vi "case_simple.vi"() -> ()   [LabVIEW 2021]
panel:
  in  "Enum":enum16{"Plus", "Minus", ""}(ring)
  in  "Numeric 13":dbl
  in  "String":string
  out "Numeric 12":dbl
  in  "Numeric 11":dbl
  in  "Numeric 10":dbl
  out "Numeric 9":dbl
  in  "Numeric 8":dbl
  in  "Numeric 7":dbl
  out "Numeric 6":dbl
  in  "Numeric 5":dbl
  in  "Numeric 4":dbl
  in  "Boolean":bool
  out "Numeric 3":dbl
  in  "Numeric 2":dbl
  in  "Numeric":dbl
  # "Method 1"
  # "Method 2"
  # "Method 3"
  # "Method 4"
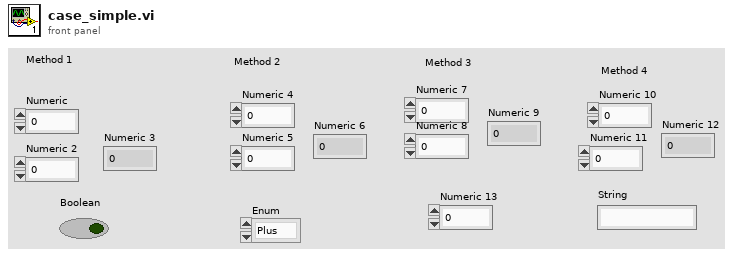
[diagram p1: front panel]
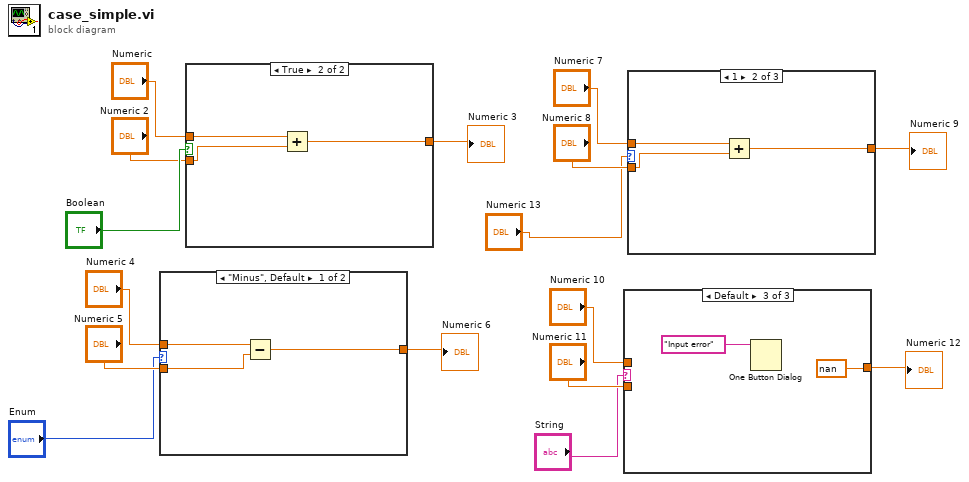
[diagram p0: block diagram]
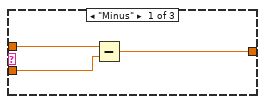
[diagram p2: hidden frame]
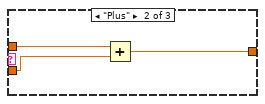
[diagram p3: hidden frame]
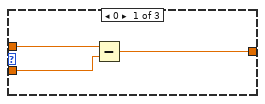
[diagram p4: hidden frame]
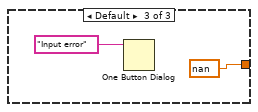
[diagram p5: hidden frame]
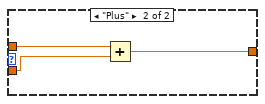
[diagram p6: hidden frame]
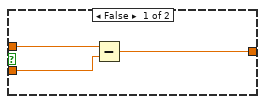
[diagram p7: hidden frame]
diagram:
  n1 = case shown="\"Minus\", Default" "Enum" {
    tunnel: [w19 w22] -> w12
    tunnel: "Numeric 4" -> [w18 w21]
    tunnel: "Numeric 5" -> [w17 w20]
    frame "Minus", Default {
      n2 = Subtract(x=w18, y=w17) -> (x-y=w19:dbl)
    }
    frame "Plus" {
      n3 = Add(x=w21, y=w20) -> (x+y=w22:dbl)
    }
  }
  "Numeric 6" <- w12
  n4 = case shown="True" "Boolean" {
    tunnel: [w25 w28] -> w15
    tunnel: "Numeric" -> [w24 w27]
    tunnel: "Numeric 2" -> [w23 w26]
    frame False {
      n5 = Subtract(x=w24, y=w23) -> (x-y=w25:dbl)
    }
    frame True {
      n6 = Add(x=w27, y=w26) -> (x+y=w28:dbl)
    }
  }
  "Numeric 3" <- w15
  n7 = case shown="Default" "String" {
    tunnel: [w31 w34 nan] -> w6
    tunnel: "Numeric 10" -> [w30 w33 _]
    tunnel: "Numeric 11" -> [w29 w32 _]
    frame "Minus" {
      n8 = Subtract(x=w30, y=w29) -> (x-y=w31:dbl)
    }
    frame "Plus" {
      n9 = Add(x=w33, y=w32) -> (x+y=w34:dbl)
    }
    frame Default {
      n10 = One Button Dialog(message="Input error") -> ()  [unwired: 1 in, 1 out]
    }
  }
  "Numeric 12" <- w6
  n11 = case shown="1" "Numeric 13" {
    tunnel: [w39 w42 nan] -> w9
    tunnel: "Numeric 7" -> [w38 w41 _]
    tunnel: "Numeric 8" -> [w37 w40 _]
    frame 0 {
      n12 = Subtract(x=w38, y=w37) -> (x-y=w39:dbl)
    }
    frame 1 {
      n13 = Add(x=w41, y=w40) -> (x+y=w42:dbl)
    }
    frame Default {
      n14 = One Button Dialog(message="Input error") -> ()  [unwired: 1 in, 1 out]
    }
  }
  "Numeric 9" <- w9
